vi "config fpga resource.vi"(0 "fpga channel in":refnum<class "FPGA Channel.lvclass">, 1 "pairs in":T2[](array[typedef]), 2 "tagbus index":i32, 3 "bitfile ref in":refnum<k20>, 4 "hardware resource":T1, 5 "error in (no error)":errorcluster) -> (14 "fpga channel out":refnum<class "FPGA Channel.lvclass">, 15 "pairs out":T2[](array[typedef]), 19 "error out":errorcluster)   [LabVIEW 2017, in "FPGA Channel.lvclass"]
uses:
  FPGA Channel.lvclass
  C:/Program Files (x86)/National Instruments/LabVIEW 2017/vi.lib/NI/Tag Bus/tag/tag descriptor.lvclass
  module/execution/ControlsMappings.ctl
  <vilib>/NI/Tag Bus/tag/Data Type.ctl
  fpga resource supported data types.ctl
  <vilib>/NI/LVFPGA Adv Session Resources/ResourceInfo.ctl
  <vilib>/NI/Tag Bus/tag/tag descriptor.lvclass/tag descriptor.ctl
  FPGA Channel.lvclass/FPGA Channel.ctl
  <vilib>/NI/Tag Bus/tag/read data type.vi
  <vilib>/NI/Tag Bus/tag/read tag name.vi
  Read FXP type.vi
  <vilib>/NI/Configuration Framework/NISE_CEF_TreeControl.lvlib
  <vilib>/NI/Tag Bus/tag/tag descriptor.lvclass
  <vilib>/NI/LVFPGA Adv Session Resources/LVFPGAAdvSessionResources.lvlib
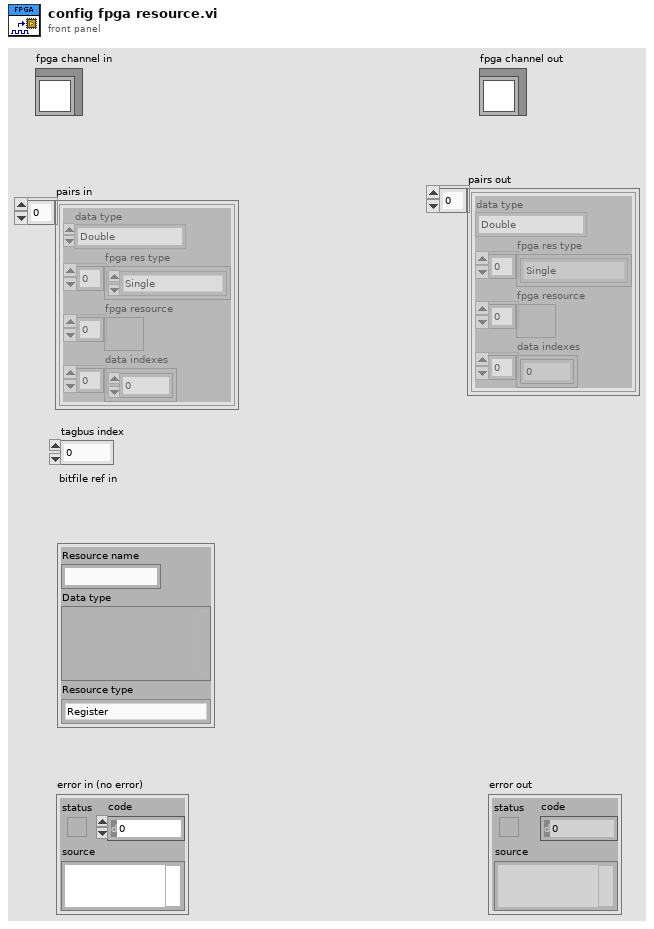
[diagram p1: front panel]
types:
  T1 = typedef "LVFPGAAdvSessionResources.lvlib/ResourceInfo.ctl" = cluster{"Resource name":string, "Data type":variant, "Resource type":enum16{"Register", "Host To Target FIFO", "Target To Host FIFO"}}
  T2 = typedef "FPGA Channel.lvclass/ControlsMappings.ctl" = cluster{"data type":T3, "fpga res type":T4[], "fpga resource":refnum<k20>[], "data indexes":i32[]}
  T3 = typedef "tag bus.lvlib/tag descriptor.lvclass/Data Type.ctl" = enum16{"Double", "Single", "I64", "I32", "I16", "I8", "U64", "U32", "U16", "U8", "Boolean", "String", "Array of Double", "Array of Single", "Array of I64", "Array of I32", "Array of I16", "Array of I8", "Array of U64", "Array of U32", "Array of U16", "Array of U8", "Array of Boolean", "Array of String"}
  T4 = typedef "FPGA Channel.lvclass/fpga resource supported data types.ctl" = enum16{"Invalid Type", "Single", "I64", "I32", "I16", "I8", "U64", "U32", "U16", "U8", "Boolean", "FXP I,20,5", "FXP I,24,5", "FXP I,24,10", "Fifo 1023,I16"}
  T5 = typedef "LVFixedPointRepBitsTypeDef.ctl" = cluster{"Signed":bool, "Word Length":u32, "Integer Word Length":i32}
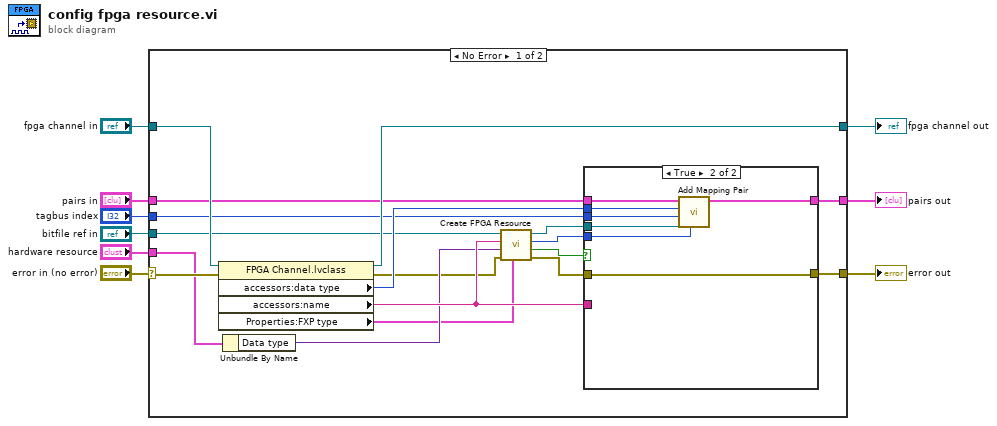
[diagram p0: block diagram]
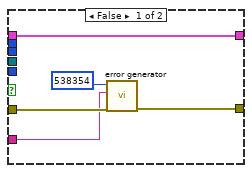
[diagram p2: hidden frame]
diagram:
  n1 = case shown="No Error" "error in (no error)" {
    selector: "error in (no error)" -> [w23 w42]
    tunnel: [w19 w42] -> w8
    tunnel: [w26 w41] -> w6
    tunnel: "fpga channel in" -> [w27 w41]
    tunnel: "pairs in" -> [w25 w40]
    tunnel: [w24 w40] -> w4
    tunnel: "bitfile ref in" -> [w15 _]
    tunnel: "tagbus index" -> [w21 _]
    tunnel: "hardware resource" -> [w20 _]
    frame No Error {
      n2 = property class="FPGA Channel.lvclass"(reference=w27, error in=w23) -> (reference out=w26:refnum<class "FPGA Channel.lvclass">, error out=w10:errorcluster, "accessors:data type"=w22:T3, "accessors:name"=w18:string, "Properties:FXP type"=w16:T5)
      n3 = Unbundle By Name(w20) -> ("Data type"=w17:variant)
      n4 = call "Create FPGA Resource.vi"("Channel FXP type"=w16, "error in (no error)"=w10, "Hardware Data type"=w17, "Resource name"=w18, "Refnum in"=w15) -> ("error out"=w11:errorcluster, "type supported"=w12:bool, "fpga res type"=w13:T4, "Refnum out"=w14:refnum<k20>)  [unwired: 3 in]
      n5 = case shown="True" w12 {
        tunnel: [w31 w38] -> w24
        tunnel: w25 -> [w31 w39]
        tunnel: w21 -> [_ w36]
        tunnel: w22 -> [_ w37]
        tunnel: [w30 w35] -> w19
        tunnel: w11 -> [w29 w35]
        tunnel: w14 -> [_ w34]
        tunnel: w13 -> [_ w33]
        tunnel: w18 -> [w28 _]
        frame False {
          n6 = call <vilib>:"error generator.vi"("error in"=w29, "append error message"=w28, "error code (0)"=538354) -> ("error out"=w30:errorcluster)  [unwired: 6 in]
        }
        frame True {
          n7 = call "Add Mapping Pair.vi"("fpga res type"=w33, "fpga resource"=w34, "data index"=w36, "data type"=w37, "pairs in"=w39) -> ("pairs out"=w38:T2[])  [unwired: 6 in]
        }
      }
    }
    frame Error {
    }
  }
  "error out" <- w8
  "fpga channel out" <- w6
  "pairs out" <- w4
